vi "acq_eeg_fin.vi"(8 "error in (no error)":errorcluster, 10 "variant in":variant, 11 "eeg_device":T1) -> (0 "error out":errorcluster)   [LabVIEW 2013]
uses:
  <vilib>/NIOSC/Address Space Node.ctl
  gui/type_def/device.ctl
  <vilib>/NI/Emotiv Toolkit/Emotiv Task.lvclass
  <vilib>/OpenBCI/Comm Protocol/Control Def/openbci_device.ctl
  <vilib>/OpenBCI/Comm Protocol/Control Def/channel_count.ctl
  gui/global_var.vi
  <vilib>/NI/LabVIEW - NeuroSky Driver/NeuroSky Driver.lvlib
  <vilib>/NIOSC/NI_OSC.lvlib
panel:
  in  "NeuroSky Task Out":T2
  in  "muse cluster":T4
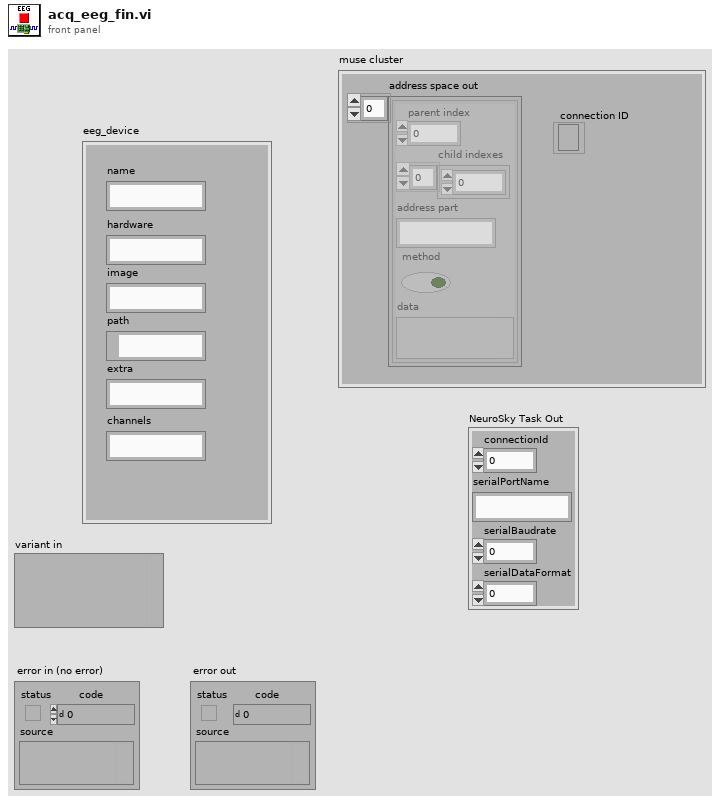
[diagram p1: front panel]
types:
  T1 = typedef "device.ctl" = cluster{"name":string, "hardware":string, "image":string, "path":path, "extra":string, "channels":string}
  T2 = cluster{"connectionId":i32, "serialPortName":string, "serialBaudrate":i32, "serialDataFormat":i32}
  T3 = typedef "NI_OSC.lvlib/Address Space Node.ctl" = cluster{"parent index":i32, "child indexes":i32[], "address part":string, "method":bool, "data":variant}
  T4 = cluster{"address space out":T3[], "connection ID":refnum<k5>}
  T5 = typedef "openbci_device.ctl" = cluster{"COM port":refnum<visa-resource-name>, "n_ch (8)":T6, "delay_tx":u32}
  T6 = typedef "channel_count.ctl" = enum16{"8 Channels", "16 Channels"}
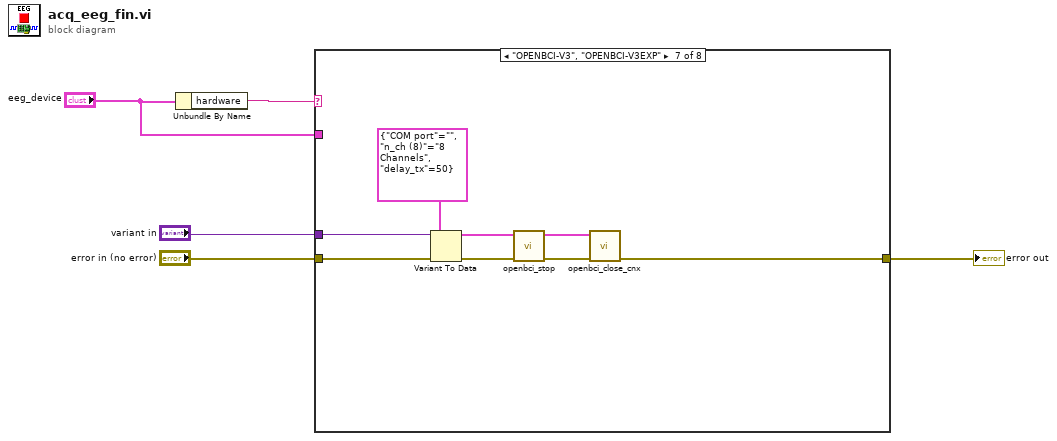
[diagram p0: block diagram]
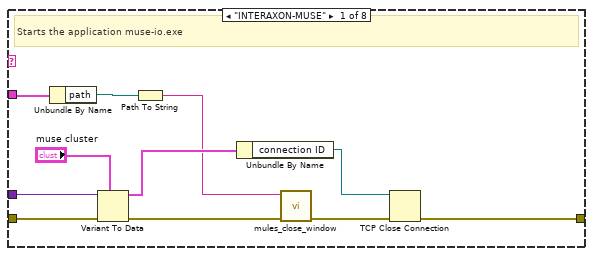
[diagram p2: hidden frame]
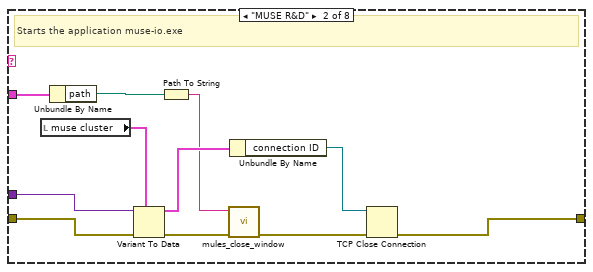
[diagram p3: hidden frame]
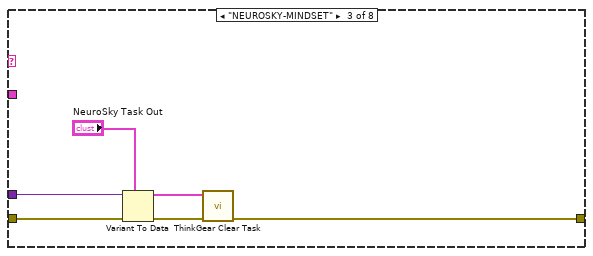
[diagram p4: hidden frame]
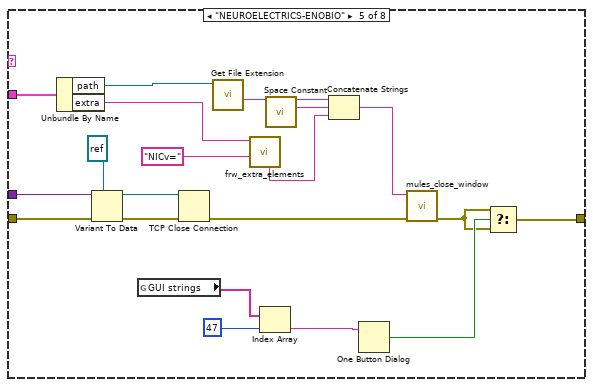
[diagram p6: hidden frame]
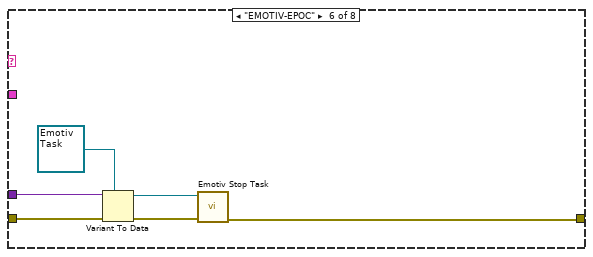
[diagram p7: hidden frame]
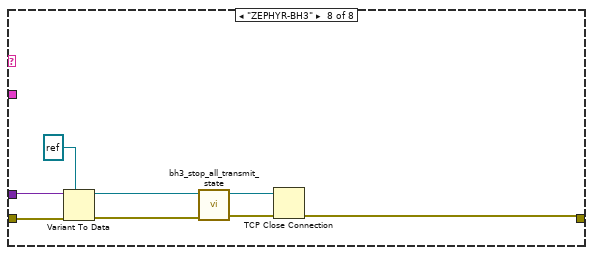
[diagram p8: hidden frame]
diagram:
  n1 = Unbundle By Name("eeg_device") -> ("hardware"=w5:string)
  n2 = case shown="\"OPENBCI-V3\", \"OPENBCI-V3EXP\"" w5 {
    tunnel: "eeg_device" -> [w11 w24 _ _ w49 _ _ _]
    tunnel: "error in (no error)" -> [w9 w22 w32 w34 w51 w58 w65 w75]
    tunnel: [w7 w20 w28 w34 w43 w56 w68 w69] -> w3
    tunnel: "variant in" -> [w15 w26 w31 _ w54 w59 w64 w74]
    frame "INTERAXON-MUSE" {
      # "Starts the application muse-io.exe"
      n3 = Unbundle By Name(w11) -> ("path"=w10:path)
      n4 = Variant To Data(error in=w9, type="muse cluster", Variant=w15) -> (data=w16:T4, error out=w6:errorcluster)
      n5 = Path To String(path=w10) -> (string=w12:string)
      n6 = Unbundle By Name(w16) -> ("connection ID"=w13:refnum<k5>)
      n7 = call "mules_close_window.vi"("error in (no error)"=w6, "IpszWindowName"=w12) -> ("sortie d'erreur"=w8:errorcluster)  [unwired: 9 in]
      n8 = TCP Close Connection(connection ID=w13, error in (no error)=w8) -> (error out=w7:errorcluster)  [unwired: 1 in, 1 out]
    }
    frame "MUSE R&D" {
      # "Starts the application muse-io.exe"
      n9 = local read "muse cluster"() -> (w21:T4)
      n10 = Unbundle By Name(w24) -> ("path"=w23:path)
      n11 = Variant To Data(error in=w22, type=w21, Variant=w26) -> (data=w27:T4, error out=w17:errorcluster)
      n12 = Path To String(path=w23) -> (string=w19:string)
      n13 = call "mules_close_window.vi"("error in (no error)"=w17, "IpszWindowName"=w19) -> ("sortie d'erreur"=w18:errorcluster)  [unwired: 9 in]
      n14 = Unbundle By Name(w27) -> ("connection ID"=w25:refnum<k5>)
      n15 = TCP Close Connection(connection ID=w25, error in (no error)=w18) -> (error out=w20:errorcluster)  [unwired: 1 in, 1 out]
    }
    frame "NEUROSKY-MINDSET" {
      n16 = Variant To Data(error in=w32, type="NeuroSky Task Out", Variant=w31) -> (data=w29:T2, error out=w33:errorcluster)
      n17 = call <vilib>:"ThinkGear Clear Task.VI"("error in"=w33, "NeuroSky Task In"=w29) -> ("error out"=w28:errorcluster)  [unwired: 9 in]
    }
    frame Default {
    }
    frame "NEUROELECTRICS-ENOBIO" {
      n18 = Unbundle By Name(w49) -> ("path"=w48:path, "extra"=w37:string)
      n19 = Variant To Data(error in=w51, type=refnum<k5> refnum ("connection ID"), Variant=w54) -> (data=w52:refnum<k5>, error out=w50:errorcluster)
      n20 = global read "global_var.vi" "GUI strings"() -> (w39:string[])
      n21 = TCP Close Connection(connection ID=w52, error in (no error)=w50) -> (error out=w44:errorcluster)  [unwired: 1 in, 1 out]
      n22 = call <vilib>:"Get File Extension.vi"("file"=w48) -> ("filename without extension"=w47:string)  [unwired: 7 in, 3 out]
      n23 = call "frw_extra_elements.vi"("single field"="NICv=" ("delimiter (Tab)"), "string"=w37) -> ("single string"=w35:string)  [unwired: 5 in, 4 out]
      n24 = Index Array(array=w39, index=47) -> (element=w38:string)
      n25 = call <vilib>:"Space Constant.vi"() -> ("String"=w46:string)
      n26 = Concatenate Strings(w47, w46, w35) -> (w45:string)
      n27 = One Button Dialog(message=w38) -> (true=w42:bool)  [unwired: 1 in]
      n28 = call "mules_close_window.vi"("error in (no error)"=w44, "IpszWindowName"=w45) -> ("sortie d'erreur"=w41:errorcluster)  [unwired: 9 in]
      n29 = Select(t=w41, s=w42, f=w41) -> (s? t:f=w43:errorcluster)
    }
    frame "EMOTIV-EPOC" {
      n30 = Variant To Data(error in=w58, type=refnum<class "Emotiv Task.lvclass"> refnum ("Emotiv Task in"), Variant=w59) -> (data=w55:refnum<class "Emotiv Task.lvclass">, error out=w57:errorcluster)
      n31 = call <vilib>:"Emotiv Stop Task.vi"("error in (no error)"=w57, "Emotiv Task in"=w55) -> ("error out"=w56:errorcluster)  [unwired: 9 in]
    }
    frame "OPENBCI-V3", "OPENBCI-V3EXP" {
      n32 = Variant To Data(error in=w65, type=T5 {"COM port"="", "n_ch (8)"=enum."8 Channels", "delay_tx"=50} ("OBCI dev in"), Variant=w64) -> (data=w62:T5, error out=w66:errorcluster)
      n33 = call <vilib>:"openbci_stop.vi"("error in (no error)"=w66, "OBCI dev in"=w62) -> ("error out"=w67:errorcluster, "OBCI dev out"=w61:T5)  [unwired: 8 in]
      n34 = call <vilib>:"openbci_close_cnx.vi"("error in (no error)"=w67, "OBCI dev in"=w61) -> ("error out"=w68:errorcluster)  [unwired: 9 in]
    }
    frame "ZEPHYR-BH3" {
      n35 = Variant To Data(error in=w75, type=refnum<k31> refnum ("bt connection ID in"), Variant=w74) -> (data=w71:refnum<k31>, error out=w72:errorcluster)
      n36 = call <vilib>:"bh3_stop_all_transmit_state.vi"("error in (no error)"=w72, "bt connection ID in"=w71) -> ("error out"=w73:errorcluster, "bt connection ID out"=w70:refnum<k31>)  [unwired: 8 in]
      n37 = TCP Close Connection(connection ID=w70, error in (no error)=w73) -> (error out=w69:errorcluster)  [unwired: 1 in, 1 out]
    }
  }
  "error out" <- w3
